vi "Data Set File Operations.vi"(8 "error in (no error)":errorcluster, 9 "Path (\"@SAVE\\mysavefile.dfl\")":string="@SAVE\\mysavefile.dfl", 10 "Operation (Save)":i32(ring) items=["Save", "Recall"], 11 "VISA resource name":refnum<visa-resource-name>) -> (0 "error out":errorcluster, 3 "VISA resource name out":refnum<visa-resource-name>)   [LabVIEW 2015, in "Rohde&Schwarz CMXP Base.lvlib"]
doc: "Stores or recalls the current instrument settings to the specified file.\n\nAttributes:\nRSCMXPBASE_ATTR_STORE_INSTRUMENT_SETTINGS\nRSCMXPBASE_ATTR_LOAD_INSTRUMENT_SETTINGS\n\nRemote-control commands:\nMMEMory:SAV\nMMEMory:RCL"
uses:
  <instrlib>/Rohde&Schwarz CMXP Base/Rohde&Schwarz CMXP Base.lvlib
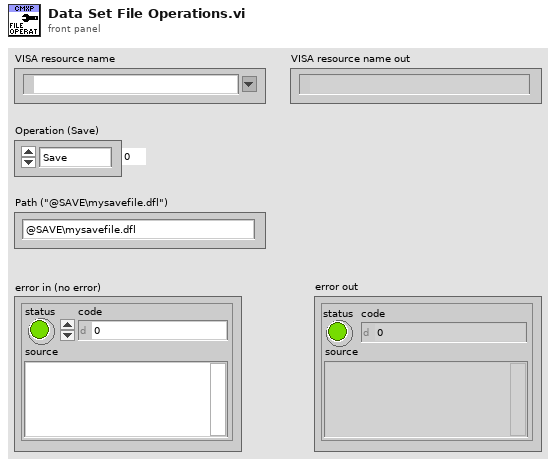
[diagram p1: front panel]
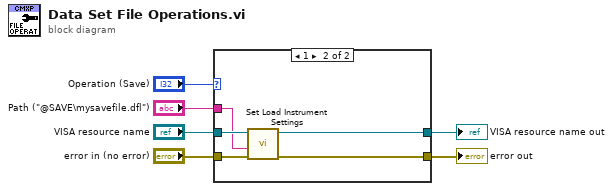
[diagram p0: block diagram]
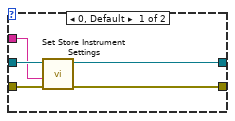
[diagram p2: hidden frame]
diagram:
  n1 = case shown="1" "Operation (Save)" {
    tunnel: "Path (\"@SAVE\\mysavefile.dfl\")" -> [w7 w12]
    tunnel: "error in (no error)" -> [w11 w16]
    tunnel: "VISA resource name" -> [w10 w15]
    tunnel: [w9 w14] -> w3
    tunnel: [w8 w13] -> w2
    frame 0, Default {
      n2 = call "Set Store Instrument Settings"("error in (no error)"=w11, "Store Instrument Settings ()"=w7, "instrument handle"=w10) -> ("error out"=w9:errorcluster, "instrument handle out"=w8:refnum<visa-resource-name>)  [unwired: 7 in]
    }
    frame 1 {
      n3 = call "Set Load Instrument Settings"("error in (no error)"=w16, "Load Instrument Settings ()"=w12, "instrument handle"=w15) -> ("error out"=w14:errorcluster, "instrument handle out"=w13:refnum<visa-resource-name>)  [unwired: 7 in]
    }
  }
  "error out" <- w3
  "VISA resource name out" <- w2
